vi "Get Events.vi"(8 "Error In":errorcluster, 11 "WebView in":refnum<class "WebView.lvclass">) -> (0 "Error Out":errorcluster, 2 "Events":T1, 3 "WebView out":refnum<class "WebView.lvclass">)   [LabVIEW 2020, in "WebView.lvclass"]
uses:
  WebView.lvclass
  WebView.lvclass/WebView.ctl
  Events--cluster.ctl
  <vilib>/sklein/WebView2/Libs/Microsoft.Web.WebView2.Core.dll
  Navigation Start Event Data--cluster.ctl
  Navigation Complete Event Data--cluster.ctl
  Source Changed Event Data--cluster.ctl
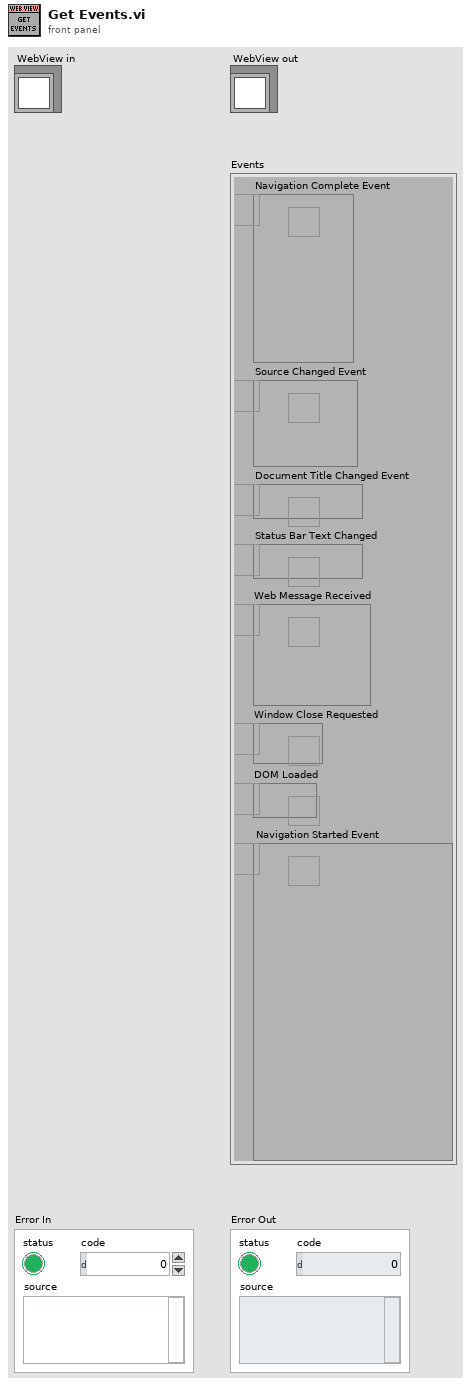
[diagram p1: front panel]
types:
  T1 = typedef "WebView.lvclass/Events--cluster.ctl" = cluster{"Navigation Complete Event":refnum<user-event>, "Source Changed Event":refnum<user-event>, "Document Title Changed Event":refnum<user-event>, "Status Bar Text Changed":refnum<user-event>, "Web Message Received":refnum<user-event>, "Window Close Requested":refnum<user-event>, "DOM Loaded":refnum<user-event>, "Navigation Started Event":refnum<user-event>}
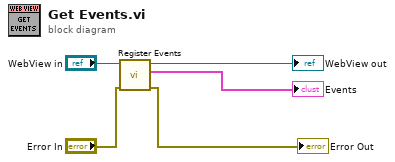
[diagram p0: block diagram]
diagram:
  n1 = call-dynamic "Register Events.vi"("Error In"="Error In", "WebView in"="WebView in") -> ("Error Out"=→"Error Out":errorcluster, "Events"=→"Events":T1, "WebView out"=→"WebView out":refnum<class "WebView.lvclass">)  [unwired: 7 in]
